vi "DAQ Data_RefreshTableValue.vi"(7 "每行显示变量个数":i32, 8 "error in":errorcluster caption="错误输入（无错误）", 9 "Data":dbl[](array[numeric]), 10 "ChannelUnits":string[](array[string]), 11 "ChannelNames":string[](array[string])) -> (0 "error out":errorcluster caption="错误输出", 2 "Table Data":string[][](array[string]))   [LabVIEW 2016]
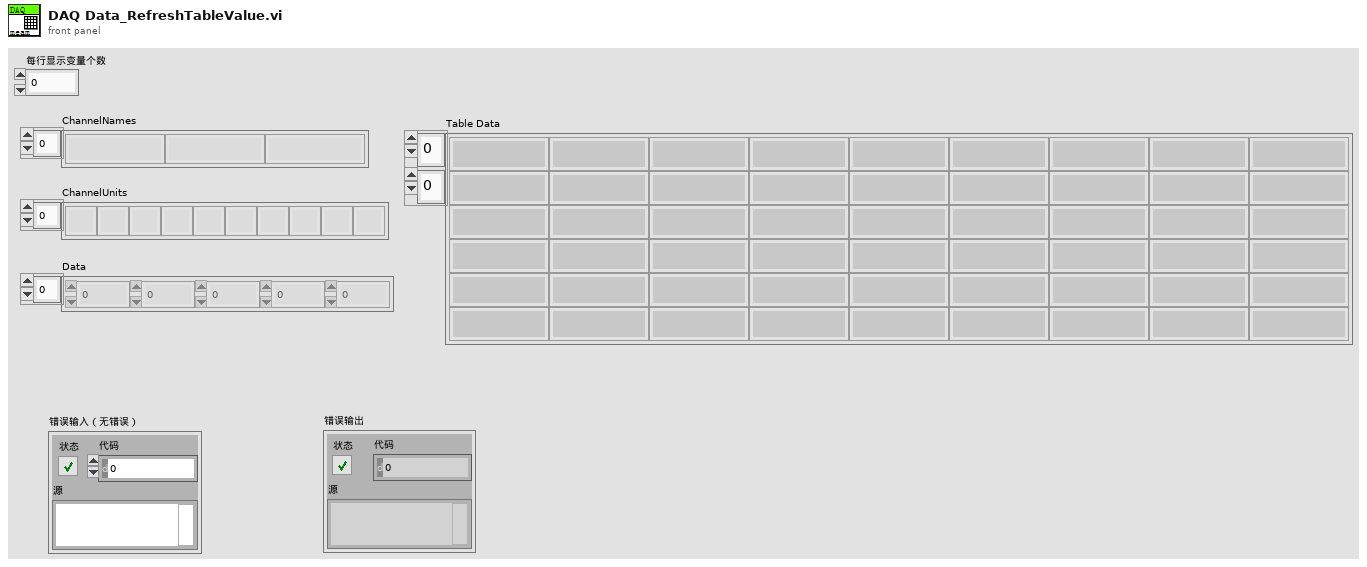
[diagram p1: front panel]
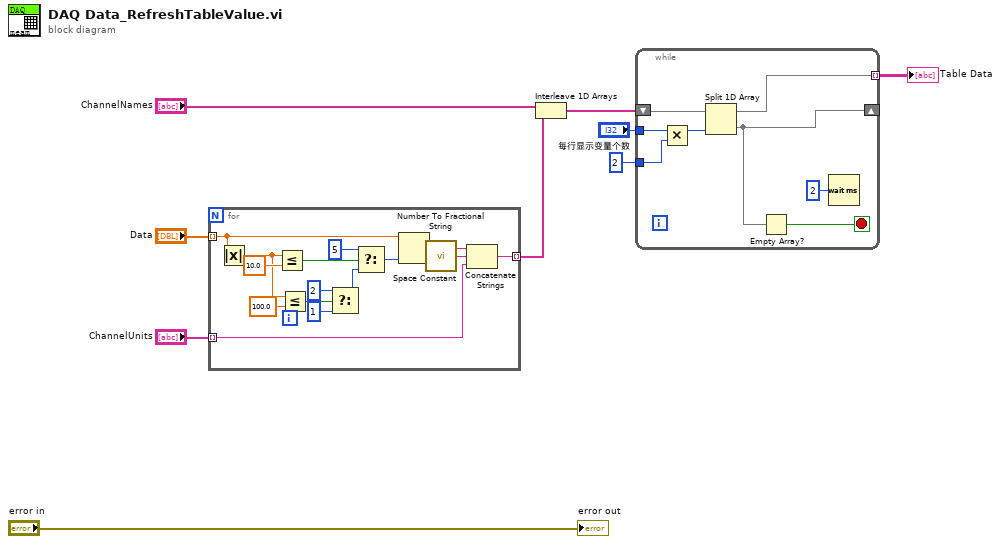
[diagram p0: block diagram]
diagram:
  n1 = for {
    tunnel: "Data" -> [w20] mode=indexing
    tunnel: "ChannelUnits" -> [w23] mode=indexing
    tunnel: [w22] -> w5 mode=indexing
    n2 = Absolute Value(x=w20) -> (abs(x)=w16:dbl)
    n3 = Less Or Equal?(x=w16, y=10.0) -> (x <= y?=w17:bool)
    n4 = Less Or Equal?(x=w16, y=100.0) -> (x <= y?=w14:bool)
    n5 = Select(t=i16 2 ("精度(6)"), s=w14, f=i16 1) -> (s? t:f=w12:i16)
    n6 = Select(t=i16 5 ("精度(6)"), s=w17, f=w12) -> (s? t:f=w10:i16)
    n7 = Number To Fractional String(number=w20, precision (6)=w10) -> (F-format string=w21:string)  [unwired: 2 in]
    n8 = call <vilib>:"Space Constant.vi"() -> ("String"=w24:string)
    n9 = Concatenate Strings(w21, w24, w23) -> (w22:string)
  }
  n10 = Interleave 1D Arrays("ChannelNames", w5) -> (w4:string[])
  n11 = while {
    shift-right: [w29] -> _
    shift-left: w4 -> [w32]
    tunnel: "每行显示变量个数" -> [w31]
    tunnel: [w30] -> w2 mode=indexing
    tunnel: 2 ("y") -> [w25]
    stop <- w28 stop-if-true
    n12 = Multiply(x=w31, y=w25) -> (x*y=w26:i32)
    n13 = Split 1D Array(array=w32, index=w26) -> (first subarray=w30:string[], second subarray=w29:string[])
    n14 = Empty Array?(array=w29) -> (empty?=w28:bool)
    n15 = Wait (ms)(milliseconds to wait=u32 2 ("等待时间（毫秒）")) -> ()  [unwired: 1 out]
  }
  "Table Data" <- w2
  "error out" <- "error in"
